vi "exercise 1.vi"() -> ()   [LabVIEW 2017]
uses:
  Pitch Array 1.ctl
  <vilib>/Analysis/coordinate.llb/Angle Range (Degree).ctl
  <vilib>/Analysis/coordinate.llb/Angle Units.ctl
  <vilib>/Analysis/coordinate.llb/Wrap Angle (scalar).vi
  <vilib>/Analysis/NI_AAL_Angle.lvlib
panel:
  out "Fan B":dbl(slide) scale=0.0..10.0
  out "Fan A":dbl(slide) scale=0.0..10.0
  in  "Power":dbl(slide) scale=0.0..100.0
  in  "Bias":dbl(slide) scale=-25.0..25.0
  out "Pitch Angle":dbl(slide)=-1.6306457677227648 scale=-80.0..80.0
  out "Absolute Travel Angle":dbl=10.26 format="%0.2f"
  out "Travel Angle":dbl(knob)=10.26 scale=0.0..360.0
  out "Elevation":dbl(slide)=-45.29166078769485 scale=-50.0..50.0
  in  "Pitch Calib":T1={"Array"=[[80.0, 4.57, 1.0, 1.0, 1.0, 1.0, 1.0, 1.0, 1.0], [70.0, 4.38, 0.0, 0.0, 0.0, 0.0, 0.0, 0.0, 0.0], [60.0, 4.22, 0.0, 0.0, 0.0, 0.0, 0.0, 0.0, 0.0], [50.0, 3.94, 0.0, 0.0, 0.0, 0.0, 0.0, 0.0, 0.0], [40.0, 3.69, 0.0, 0.0, 0.0, 0.0, 0.0, 0.0, 0.0], [30.0, 3.36, 0.0, 0.0, 0.0, 0.0, 0.0, 0.0, 0.0], [20.0, 3.01, 0.0, 0.0, 0.0, 0.0, 0.0, 0.0, 0.0], [10.0, 2.73, 0.0, 0.0, 0.0, 0.0, 0.0, 0.0, 0.0], [0.0, 2.36, 0.0, 0.0, 0.0, 0.0, 0.0, 0.0, 0.0], [-10.0, 2.15, 0.0, 0.0, 0.0, 0.0, 0.0, 0.0, 0.0], [-20.0, 1.79, 0.0, 0.0, 0.0, 0.0, 0.0, 0.0, 0.0], [-30.0, 1.38, 0.0, 0.0, 0.0, 0.0, 0.0, 0.0, 0.0], [-40.0, 1.12, 0.0, 0.0, 0.0, 0.0, 0.0, 0.0, 0.0], [-50.0, 0.92, 0.0, 0.0, 0.0, 0.0, 0.0, 0.0, 0.0], [-60.0, 0.7, 0.0, 0.0, 0.0, 0.0, 0.0, 0.0, 0.0], [-70.0, 0.53, 0.0, 0.0, 0.0, 0.0, 0.0, 0.0, 0.0], [-80.0, 0.39, 0.0, 0.0, 0.0, 0.0, 0.0, 0.0, 0.0]], "Operation"=FALSE}
  in  "stop":bool
  # "Calibration\nMode"
  # "Operating\nMode"
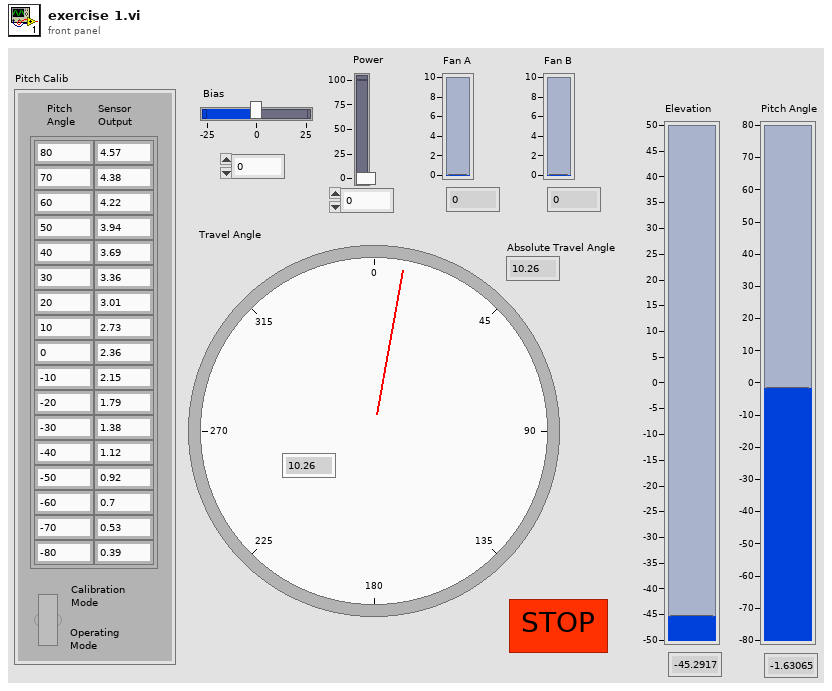
[diagram p1: front panel]
types:
  T1 = typedef "Pitch Array 1.ctl" = cluster{"Array":dbl[][], "Operation":bool}
  T2 = cluster{"AI Task":refnum<k21>, "Ctr0 Task":refnum<k21>, "Ao Task":refnum<k21>, "DO Task":refnum<k21>}
  T3 = typedef "NI_AAL_Angle.lvlib/Angle Units.ctl" = i32
  T4 = typedef "NI_AAL_Angle.lvlib/Angle Range (Degree).ctl" = u16
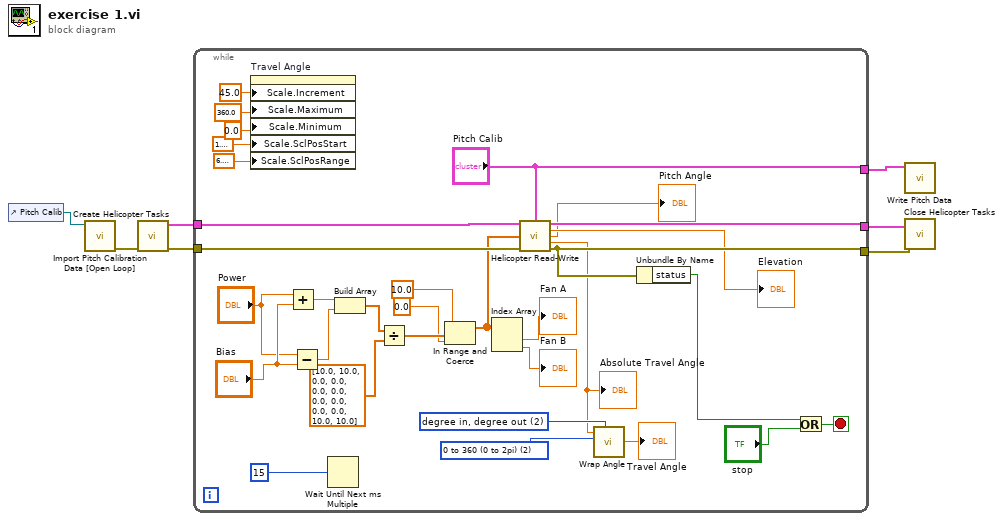
[diagram p0: block diagram]
diagram:
  n1 = control-ref of="Pitch Calib"() -> (w2:refnum<vi>)
  n2 = call "Import Pitch Calibration Data [Open Loop].vi"("Pitch Data Ref"=w2) -> ("Error Out"=w3:errorcluster)  [unwired: 10 in]
  n3 = call "Create Helicopter Tasks.vi"("Error In"=w3) -> ("Error Out"=w6:errorcluster, "Hellicopter Tasks Output"=w7:T2)  [unwired: 5 in]
  n4 = while {
    tunnel: w7 -> [w37]
    tunnel: w6 -> [w36]
    tunnel: [w34] -> w5
    tunnel: [w35] -> w4
    tunnel: ["Pitch Calib"] -> w1
    stop <- w39 stop-if-true
    w23 = T3 2 items=["radian in, radian out", "radian in, degree out", "degree in, degree out", "degree in, radian out"] ("angle units")
    w24 = T4 2 items=["none", "-180 to 180 (-pi to pi)", "0 to 360 (0 to 2pi)"] ("angle range")
    n5 = property on="Travel Angle" class="Knob (strict)"("Scale.Increment"=45.0 ("Scale.Range:Increment"), "Scale.Maximum"=360.0 ("Scale.Range:Maximum"), "Scale.Minimum"=0.0 ("Scale.Range:Minimum"), "Scale.SclPosStart"=1.5707963267948966, "Scale.SclPosRange"=6.283185307179586) -> ()  [unwired: 2 in, 2 out]
    n6 = Add(x="Power", y="Bias") -> (x+y=w15:dbl)
    n7 = Subtract(x="Power", y="Bias") -> (x-y=w18:dbl)
    n8 = Wait Until Next ms Multiple(millisecond multiple=u32 15) -> ()  [unwired: 1 out]
    n9 = Build Array(w15, w18) -> (w19:dbl[])
    n10 = Divide(x=w19, y=dbl[] [10.0, 10.0, 0.0, 0.0, 0.0, 0.0, 0.0, 0.0, 0.0, 0.0, 10.0, 10.0]) -> (x/y=w14:dbl[])
    n11 = In Range and Coerce(upper limit=10.0, x=w14, lower limit=0.0) -> (coerced(x)=w8:dbl[])  [unwired: 1 out]
    n12 = Index Array(array=w8) -> (element #1=→"Fan A":dbl, element #2=→"Fan B":dbl)  [unwired: 2 in]
    n13 = call "Helicopter Read-Write.vi"("Hellicopter Tasks Input"=w37, "Pitch Calib"="Pitch Calib", "Fan Input"=w8, "Error In"=w36) -> ("Hellicopter Tasks Output"=w35:T2, "Elevation"=→"Elevation":dbl, "Pitch"=→"Pitch Angle":dbl, "Travel"=w21:dbl, "Error Out"=w34:errorcluster)  [unwired: 7 in]
    "Absolute Travel Angle" <- w21
    n14 = call-poly <vilib>:"Wrap Angle.vi"("angle units"=w23, "angle range"=w24, "angle in"=w21) -> ("angle out"=→"Travel Angle":dbl)  [unwired: 7 in, 1 out]
    n15 = Unbundle By Name(w34) -> ("status"=w33:bool)
    n16 = Or(x=w33, y="stop") -> (x .or. y?=w39:bool)
  }
  n17 = call "Write Pitch Data.vi"("Pitch Calib"=w1) -> ()  [unwired: 11 in]
  n18 = call "Close Helicopter Tasks.vi"("Error In"=w5, "Hellicopter Tasks Input 2"=w4) -> ()  [unwired: 9 in, 1 out]
